vi "LEDdiy.vi"() -> ()   [LabVIEW 2015]
panel:
  out "appended array 2":bool[](array[boolean])
  out "appended array":bool[](array[boolean])
  in  "stop":bool
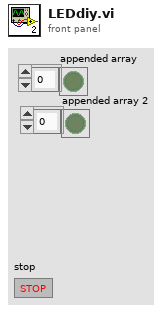
[diagram p1: front panel]
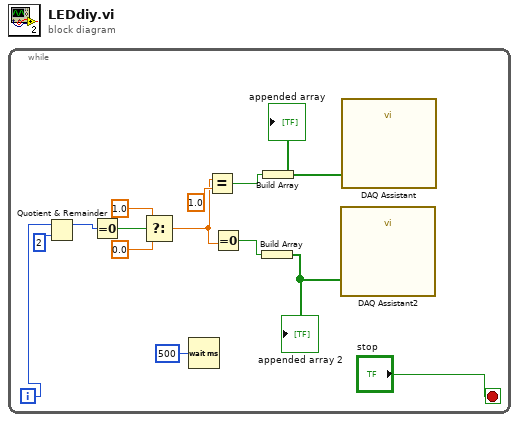
[diagram p0: block diagram]
diagram:
  n1 = while {
    i -> [w4]
    stop <- "stop" stop-if-true
    n2 = Quotient & Remainder(x=w4, y=2) -> (x-y*floor(x/y)=w2:i32)  [unwired: 1 out]
    n3 = Equal To 0?(x=w2) -> (x = 0?=w13:bool)
    n4 = Select(t=1.0, s=w13, f=0.0) -> (s? t:f=w9:dbl)
    n5 = Wait (ms)(milliseconds to wait=u32 500) -> ()  [unwired: 1 out]
    n6 = Equal?(x=w9, y=1.0) -> (x = y?=w8:bool)
    n7 = Equal To 0?(x=w9) -> (x = 0?=w6:bool)
    n8 = Build Array(w6) -> (w5:bool[])
    "appended array 2" <- w5
    n9 = Build Array(w8) -> (w7:bool[])
    "appended array" <- w7
    n10 = call "DAQ Assistant2"("data"=w5) -> ()  [unwired: 17 in, 2 out]
    n11 = call "DAQ Assistant"("data"=w7) -> ()  [unwired: 17 in, 2 out]
  }
